vi "AnalogSettings.vi"(1 "Get/Set":bool, 2 "Analog Settings (input)":T1={"PCI 671x Device Number"=1, "Samples per Unit"=10}) -> (0 "Analog Settings (output)":T1={"PCI 671x Device Number"=2, "Samples per Unit"=10})   [LabVIEW 2009]
uses:
  AnalogSettings.ctt
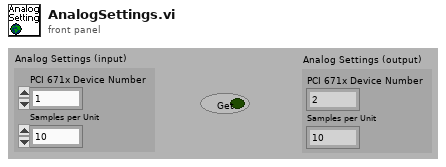
[diagram p1: front panel]
types:
  T1 = typedef "AnalogSettings.ctt" = cluster{"PCI 671x Device Number":u32, "Samples per Unit":u32}
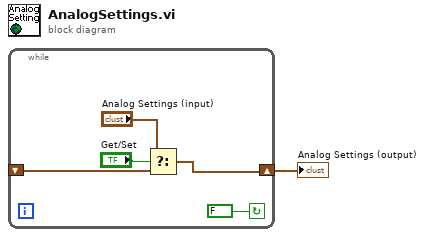
[diagram p0: block diagram]
diagram:
  n1 = while {
    shift-right: [w4] -> w1
    shift-left: _ -> [w5]
    stop <- FALSE continue-if-true
    n2 = Select(t="Analog Settings (input)", s="Get/Set", f=w5) -> (s? t:f=w4:T1)
  }
  "Analog Settings (output)" <- w1
